vi "How Search and Replace Operation In Array.vi"() -> ()   [LabVIEW 2020]
panel:
  in  "Cluster 3":T1 {"Small Cluster 3"."Slide Value" scale=0.0..10.0; "Cluster Modified"."Slide 2" scale=0.0..10.0; "Cluster"."Slide" scale=0.0..10.0}
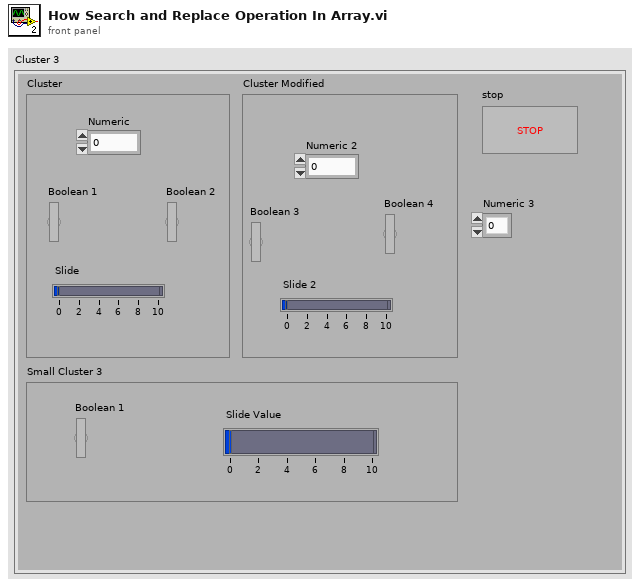
[diagram p1: front panel]
types:
  T1 = cluster{"Cluster":cluster{"Numeric":dbl, "Boolean 1":bool, "Boolean 2":bool, "Slide":dbl}, "Cluster Modified":cluster{"Numeric 2":dbl, "Boolean 3":bool, "Boolean 4":bool, "Slide 2":dbl}, "stop":bool, "Numeric 3":dbl, "Small Cluster 3":cluster{"Boolean 1":bool, "Slide Value":dbl}}
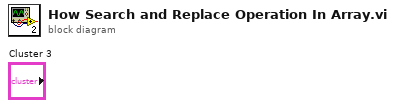
[diagram p0: block diagram]
diagram:
